vi "startReadManual.vi"(8 "error in (no error)":errorcluster, 10 "ElectrometerController in":refnum<class "ElectrometerController.lvclass">, 11 "ReadyState in":refnum<class "ReadyState.lvclass">) -> (0 "error out":errorcluster, 2 "ElectrometerController out":refnum<class "ElectrometerController.lvclass">, 3 "ReadyState out":refnum<class "ReadyState.lvclass">)   [LabVIEW 2016, in "ReadyState.lvclass"]
uses:
  ReadyState.lvclass
  ElectrometerController/ElectrometerController.lvclass
  internalState.ctl
  State.lvclass
  Electrometer.lvclass
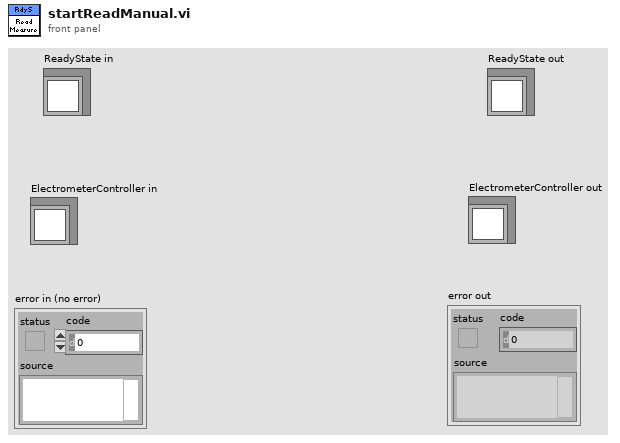
[diagram p1: front panel]
types:
  T1 = typedef "Electrometer.lvclass/internalState.ctl" = enum16{"Ready", "Configuring", "ManualReading", "UntilIntensityReading", "SetDurationReading"}
  T2 = typedef "Electrometer.lvclass/Modes.ctl" = enum16{"Current", "Charge", "Voltage", "Resistance"}
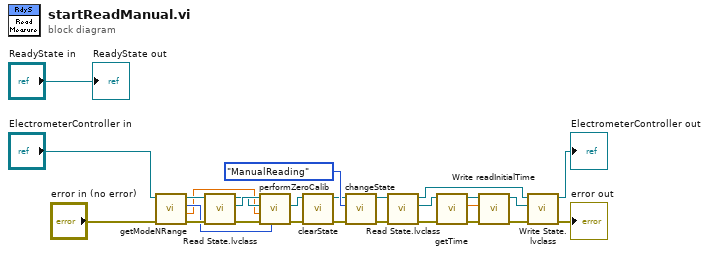
[diagram p0: block diagram]
diagram:
  n1 = call-dynamic "getModeNRange.vi"("error in (no error)"="error in (no error)", "ElectrometerController in"="ElectrometerController in") -> ("error out"=w16:errorcluster, "Input Range"=w14:dbl, "Mode"=w15:T2, "ElectrometerController out"=w17:refnum<class "ElectrometerController.lvclass">)  [unwired: 6 in]
  n2 = call-dynamic "Read State.lvclass.vi"("error in (no error)"=w16, "ElectrometerController in"=w17) -> ("error out"=w18:errorcluster, "State.lvclass"=w20:refnum<class "State.lvclass">, "ElectrometerController out"=w19:refnum<class "ElectrometerController.lvclass">)  [unwired: 7 in]
  n3 = call-dynamic "performZeroCalib.vi"("Mode"=w15, "error in (no error)"=w18, "Input Range"=w14, "ElectrometerController in"=w19, "State in"=w20) -> ("error out"=w8:errorcluster, "ElectrometerController out"=w11:refnum<class "ElectrometerController.lvclass">)  [unwired: 3 in, 2 out]
  n4 = call "clearState.vi"("error in (no error)"=w8, "ElectrometerController in"=w11) -> ("error out"=w9:errorcluster, "ElectrometerController out"=w10:refnum<class "ElectrometerController.lvclass">)  [unwired: 8 in]
  n5 = call "changeState.vi"("error in (no error)"=w9, "State"=internalState."ManualReading", "ElectrometerController in"=w10) -> ("error out"=w5:errorcluster, "ElectrometerController out"=w4:refnum<class "ElectrometerController.lvclass">)  [unwired: 7 in]
  n6 = call-dynamic "Read State.lvclass.vi"("error in (no error)"=w5, "ElectrometerController in"=w4) -> ("error out"=w1:errorcluster, "State.lvclass"=w2:refnum<class "State.lvclass">, "ElectrometerController out"=w3:refnum<class "ElectrometerController.lvclass">)  [unwired: 7 in]
  n7 = call-dynamic "getTime.vi"("error in (no error)"=w1, "State in"=w2) -> ("error out"=w23:errorcluster, "relative seconds"=w24:dbl, "State out"=w22:refnum<class "State.lvclass">)  [unwired: 7 in]
  n8 = call-dynamic "Write readInitialTime.vi"("error in (no error)"=w23, "readInitialTime"=w24, "State in"=w22) -> ("error out"=w25:errorcluster, "State out"=w26:refnum<class "State.lvclass">)  [unwired: 7 in]
  n9 = call-dynamic "Write State.lvclass.vi"("error in (no error)"=w25, "State.lvclass"=w26, "ElectrometerController in"=w3) -> ("error out"=→"error out":errorcluster, "ElectrometerController out"=→"ElectrometerController out":refnum<class "ElectrometerController.lvclass">)  [unwired: 7 in]
  "ReadyState out" <- "ReadyState in"
